vi "expressVI.vi"() -> ()   [LabVIEW 2017]
panel:
  in  "stop":bool
  in  "rate":dbl=1000.0
  out "Waveform Graph":dynamicdata(graph)
  in  "timeout (s)":dbl=10.0 format="%0.2f"
  out "error out":errorcluster
  in  "number of samples":i32=1000
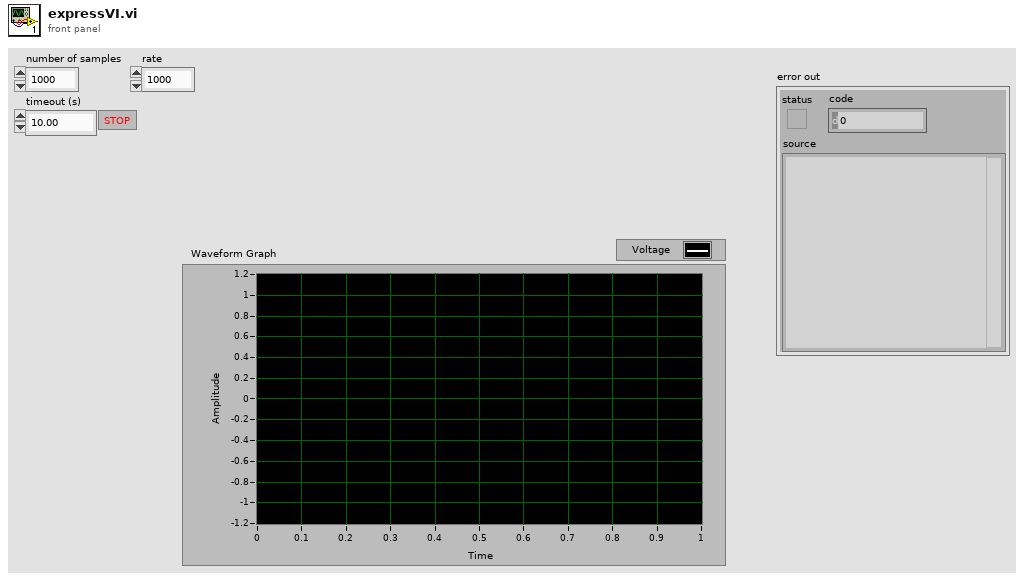
[diagram p1: front panel]
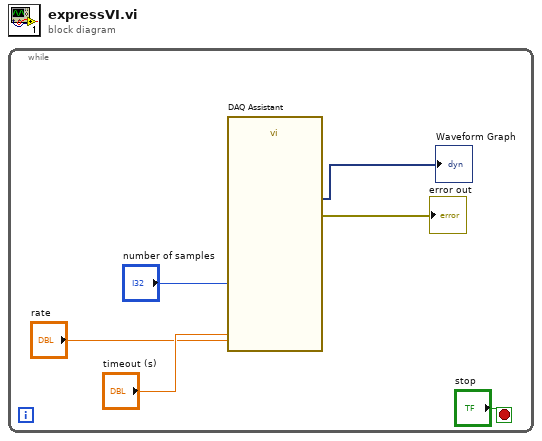
[diagram p0: block diagram]
diagram:
  n1 = while {
    stop <- "stop" stop-if-true
    n2 = call "DAQ Assistant"("rate"="rate", "number of samples"="number of samples", "timeout (s)"="timeout (s)") -> ("data"=→"Waveform Graph":dynamicdata, "error out"=→"error out":errorcluster)  [unwired: 14 in, 1 out]
  }
